vi "Get Magnet Field.vi"(6 "Axis":T1, 8 "error in (no error)":errorcluster, 11 "instrument.PPMS in":refnum<class "instrument.PPMS3.lvclass">) -> (0 "error out":errorcluster, 1 "Status":variant, 2 "B Field (T)":dbl, 3 "instrument.PPMS out":refnum<class "instrument.PPMS3.lvclass">, 4 "Finished?":bool)   [LabVIEW 2016, in "instrument.PPMS3.lvclass"]
uses:
  instrument.PPMS3.lvclass
  <userlib>/LevyLab/Levylab Instruments/Instrument Types/Cryostat/Typedefs/Magnet Axis--Enum.ctl
  Typedefs/PPMS.Magnet Status--cluster.ctl
  Typedefs/PPMS.Commands-enum.ctl
  <userlib>/LevyLab/Levylab Instruments/Instrument Types/Cryostat/Instrument.Cryostat.lvclass
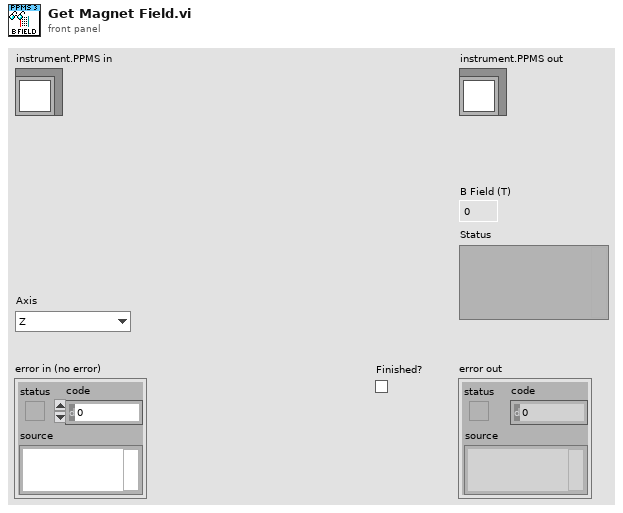
[diagram p1: front panel]
types:
  T1 = typedef "Instrument.Cryostat.lvclass/Magnet Axis--Enum.ctl" = enum16{"Z", "X", "Y"}
  T2 = typedef "instrument.PPMS3.lvclass/PPMS.Commands-enum.ctl" = enum16{"Get Magnet Field", "Get Helium Level", "Get Temperature", "Set Magnet Field", "Set Temperature", "getAll"}
  T3 = typedef "instrument.PPMS3.lvclass/PPMS.Magnet Status--cluster.ctl" = cluster{"Field (Oe)":dbl, "Magnet Status":string}
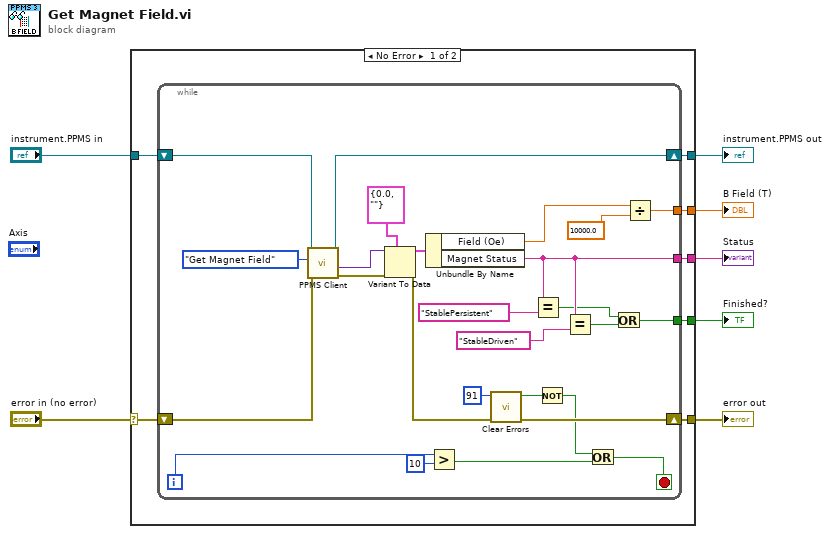
[diagram p0: block diagram]
diagram:
  n1 = case shown="No Error" "error in (no error)" {
    selector: "error in (no error)" -> [w9 w42]
    tunnel: [w14 w42] -> w7
    tunnel: [w13 w41] -> w6
    tunnel: "instrument.PPMS in" -> [w12 w41]
    tunnel: [w11 _] -> w4
    tunnel: [w10 _] -> w3
    tunnel: [w8 _] -> w1
    frame No Error {
      n2 = while {
        tunnel: [w21] -> w11
        tunnel: [w35] -> w10
        shift-right: [w29] -> w14
        shift-left: w9 -> [w39]
        shift-right: [w38] -> w13
        shift-left: w12 -> [w37]
        tunnel: [w17] -> w8
        i -> [w23]
        stop <- w24 stop-if-true
        n3 = call "PPMS Client.vi"("error in (no error)"=w39, "Command"=PPMS.Commands-enum."Get Magnet Field", "instrument.PPMS in"=w37) -> ("error out"=w32:errorcluster, "Data out"=w33:variant, "instrument.PPMS out"=w38:refnum<class "instrument.PPMS3.lvclass">)  [unwired: 5 in, 1 out]
        n4 = Variant To Data(error in=w32, type=T3 {"Field (Oe)"=0.0, "Magnet Status"=""} ("cluster"), Variant=w33) -> (data=w34:T3, error out=w40:errorcluster)
        n5 = Unbundle By Name(w34) -> ("Field (Oe)"=w30:dbl, "Magnet Status"=w21:string)
        n6 = Greater?(x=w23, y=10) -> (0:w26:bool)
        n7 = call <vilib>:"Clear Errors.vi"("error in (no error)"=w40, "specific error code to clear (0: all)"=91) -> ("error out"=w29:errorcluster, "specific error cleared?"=w25:bool)  [unwired: 4 in]
        n8 = Equal?(x=w21, y="StablePersistent") -> (x = y?=w19:bool)
        n9 = Not(x=w25) -> (.not. x?=w16:bool)
        n10 = Equal?(x=w21, y="StableDriven") -> (x = y?=w18:bool)
        n11 = Or(x=w16, y=w26) -> (x .or. y?=w24:bool)
        n12 = Or(x=w19, y=w18) -> (x .or. y?=w17:bool)
        n13 = Divide(x=w30, y=10000.0) -> (x/y=w35:dbl)
      }
    }
    frame Error {
    }
  }
  "error out" <- w7
  "instrument.PPMS out" <- w6
  "B Field (T)" <- w3
  "Status" <- w4
  "Finished?" <- w1
